vi "GetEncoderDistance (1).vi"(8 "Encoder Count":i32, 10 "Resolution (Counts per rev)":dbl, 11 "Lead Screw Lead (mm/rev)":dbl) -> (0 "Distance from origin (mm)":dbl)   [LabVIEW 2013]
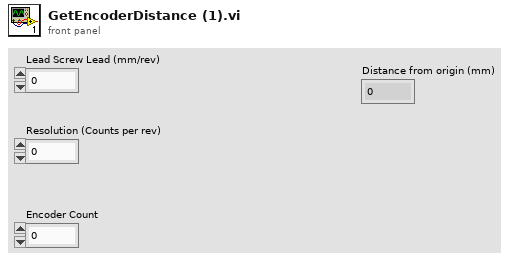
[diagram p1: front panel]
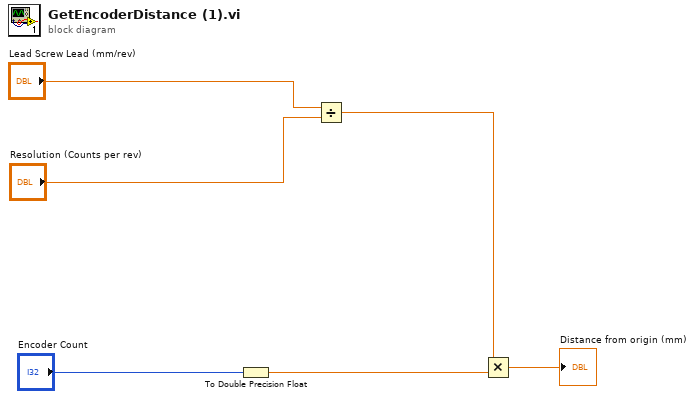
[diagram p0: block diagram]
diagram:
  n1 = To Double Precision Float(number="Encoder Count") -> (double precision float=w3:dbl)
  n2 = Divide(x="Lead Screw Lead (mm/rev)", y="Resolution (Counts per rev)") -> (x/y=w2:dbl)
  n3 = Multiply(x=w2, y=w3) -> (x*y=→"Distance from origin (mm)":dbl)
